vi "Update.vi"(7 "Adresse":T1, 8 "error in (no error)":errorcluster, 11 "VISA resource name":refnum<visa-resource-name>) -> (0 "error out":errorcluster, 3 "VISA resource name out":refnum<visa-resource-name>)   [LabVIEW 2023, in "TCxxxx.lvlib"]
doc: "This VI programs a value written before with one of the Write functions into the EEProm.\n\n\nInput\n\n- Adresse [ENUM]: this is the adress at which the function performs the read\n\n\n\nOutput:\n\n- \n\n\n\n\nLast Revision: 1.0\nDate: 19.12.2016\n\nTameq Schweiz GmbH\nPeter Wilhelm\nDorfstrasse 59\nCH-5306 Tegerfelden"
uses:
  TCxxxx.lvlib
  Controls/Adresse.ctl
panel:
  in  "Parameter [-32768 ... 0 ... 32767]":i16
  in  "Befehl [0 ... 65535]":u16
  out "Read Buffer":string
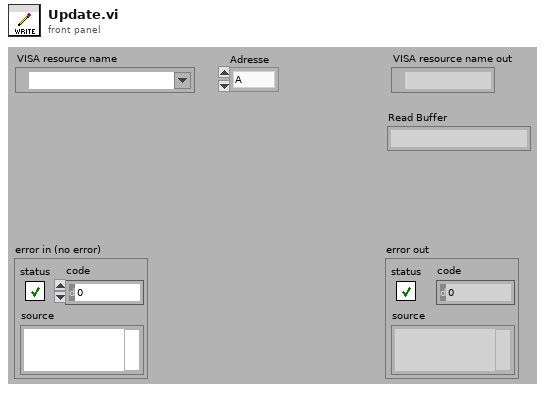
[diagram p1: front panel]
types:
  T1 = typedef "Adresse.ctl" = enum16{"A", "B", "C", "D", "E", "F", "G", "H", "I", "J", "K", "L", "M", "N", "O", "P", "Q", "R", "S", "T", "U", "V", "W", "X", "Y", "Z"}
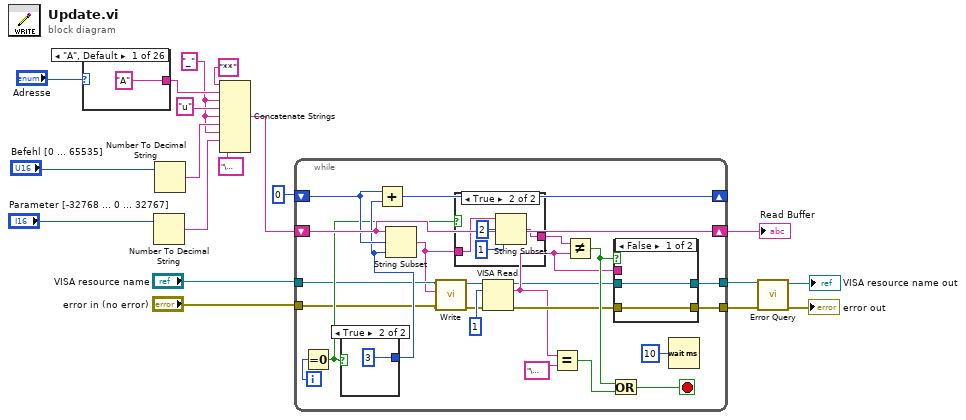
[diagram p0: block diagram]
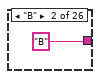
[diagram p2: hidden frame]
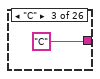
[diagram p3: hidden frame]
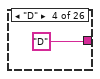
[diagram p4: hidden frame]
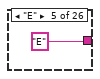
[diagram p5: hidden frame]
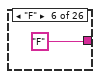
[diagram p6: hidden frame]
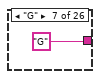
[diagram p7: hidden frame]
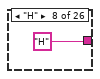
[diagram p8: hidden frame]
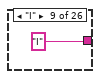
[diagram p9: hidden frame]
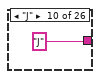
[diagram p10: hidden frame]
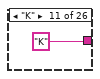
[diagram p11: hidden frame]
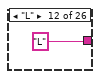
[diagram p12: hidden frame]
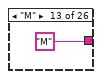
[diagram p13: hidden frame]
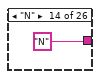
[diagram p14: hidden frame]
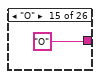
[diagram p15: hidden frame]
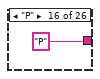
[diagram p16: hidden frame]
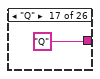
[diagram p17: hidden frame]
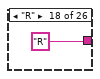
[diagram p18: hidden frame]
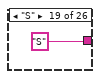
[diagram p19: hidden frame]
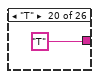
[diagram p20: hidden frame]
diagram:
  w11 = "_"
  n1 = case shown="\"A\", Default" "Adresse" {
    tunnel: ["A" "B" "C" "D" "E" "F" "G" "H" "I" "J" "K" "L" "M" "N" "O" "P" "Q" "R" "S" "T" "U" "V" "W" "X" "Y" "Z"] -> w18
    frame "A", Default {
    }
    frame "B" {
    }
    frame "C" {
    }
    frame "D" {
    }
    frame "E" {
    }
    frame "F" {
    }
    frame "G" {
    }
    frame "H" {
    }
    frame "I" {
    }
    frame "J" {
    }
    frame "K" {
    }
    frame "L" {
    }
    frame "M" {
    }
    frame "N" {
    }
    frame "O" {
    }
    frame "P" {
    }
    frame "Q" {
    }
    frame "R" {
    }
    frame "S" {
    }
    frame "T" {
    }
    frame "U" {
    }
    frame "V" {
    }
    frame "W" {
    }
    frame "X" {
    }
    frame "Y" {
    }
    frame "Z" {
    }
  }
  n2 = Number To Decimal String(number="Parameter [-32768 ... 0 ... 32767]") -> (decimal integer string=w16:string)  [unwired: 1 in]
  n3 = Number To Decimal String(number="Befehl [0 ... 65535]") -> (decimal integer string=w17:string)  [unwired: 1 in]
  n4 = Concatenate Strings("**", w18, w11, "u", w11, w17, w11, w16, "\u0015") -> (w15:string)
  n5 = while {
    tunnel: [w55] -> w9
    tunnel: [w52] -> w10
    tunnel: "error in (no error)" -> [w49]
    tunnel: "VISA resource name" -> [w51]
    shift-right: [w68] -> w3
    shift-left: w15 -> [w68]
    shift-right: [w62] -> _
    shift-left: 0 -> [w64]
    i -> [w65]
    stop <- w60 stop-if-true
    n6 = Equal To 0?(x=w65) -> (x = 0?=w59:bool)
    n7 = case shown="True" w59 {
      tunnel: [1 3] -> w63
      frame False {
      }
      frame True {
      }
    }
    n8 = Add(x=w64, y=w63) -> (x+y=w62:i32)
    n9 = String Subset(string=w68, offset (0)=w64, length (rest)=w63) -> (substring=w50:string)
    n10 = call "Write.vi"("error in (no error)"=w49, "Write Buffer"=w50, "VISA resource name"=w51) -> ("error out"=w48:errorcluster, "VISA resource name out"=w47:refnum<visa-resource-name>)  [unwired: 6 in, 1 out]
    n11 = case shown="True" w59 {
      tunnel: w50 -> [w76 w80]
      tunnel: [w76 w78] -> w58
      frame False {
      }
      frame True {
        n12 = String Subset(string=w80, offset (0)=2, length (rest)=1 ("length (rest)")) -> (substring=w78:string)
      }
    }
    n13 = VISA Read(VISA resource name=w47, byte count=1, error in (no error)=w48) -> (VISA resource name out=w53:refnum<visa-resource-name>, read buffer=w54:string, error out=w56:errorcluster)  [unwired: 1 out]
    n14 = Equal?(x=w54, y="\u0015") -> (x = y?=w61:bool)
    n15 = Not Equal?(x=w58, y=w54) -> (x != y?=w57:bool)
    n16 = Or(x=w57, y=w61) -> (x .or. y?=w60:bool)
    n17 = case shown="False" w57 {
      tunnel: w56 -> [w70 w73]
      tunnel: [w70 w71] -> w55
      tunnel: w54 -> [_ w75]
      tunnel: w53 -> [w69 w74]
      tunnel: [w69 w72] -> w52
      frame False {
      }
      frame True {
        n18 = call "GetStatus.vi"("error in"=w73, "Status"=w75, "VISA resource name"=w74) -> ("error out"=w71:errorcluster, "VISA resource name out"=w72:refnum<visa-resource-name>)  [unwired: 7 in]
      }
    }
    n19 = Wait (ms)(milliseconds to wait=u32 10) -> ()  [unwired: 1 out]
  }
  "Read Buffer" <- w3
  n20 = call "Error Query.vi"("error in (no error)"=w9, "VISA resource name"=w10) -> ("error out"=→"error out":errorcluster, "VISA resource name out"=→"VISA resource name out":refnum<visa-resource-name>)  [unwired: 8 in]
